vi "SRV_Parse VI Name for Version Number.vi"(7 "VI Name":string) -> (8 "Version Number":i32)   [LabVIEW 2009]
doc: "Returns the number at the end of a VI name that precedes the \".vi\".\n\n\nAuthor: Mike Schultz - Logic PD"
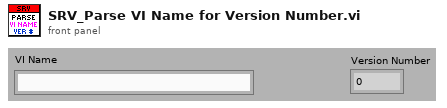
[diagram p1: front panel]
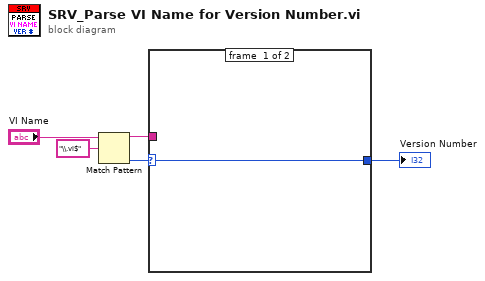
[diagram p0: block diagram]
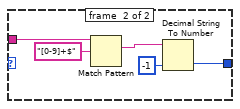
[diagram p2: hidden frame]
diagram:
  n1 = Match Pattern(string="VI Name", regular expression="\\.vi$") -> (before substring=w2:string, offset past match=w3:i32)  [unwired: 1 in, 2 out]
  n2 = case shown="Default" w3 {
    selector: w3 -> [w6 _]
    tunnel: w2 -> [_ w10]
    tunnel: [w6 w7] -> w1
    frame #0 {
    }
    frame #1 {
      n3 = Match Pattern(string=w10, regular expression="[0-9]+$") -> (match substring=w9:string)  [unwired: 1 in, 3 out]
      n4 = Decimal String To Number(string=w9, default (0L)=-1 ("default (0 I32)")) -> (number=w7:i32)  [unwired: 1 in, 1 out]
    }
  }
  "Version Number" <- w1
